vi "Connection Loop.vi"(8 "error in (no error)":errorcluster, 11 "TCP Comm":T2) -> (0 "error out":errorcluster)   [LabVIEW 2020, in "TinyTCP.lvlib"]
uses:
  TinyTCP.lvlib
  Instance.ctl
  Ref Data.ctl
  State.ctl
panel:
  out "Certificate DN":string
  out "TLS Enabled":bool
  out "Server":bool
  out "Port":u16
  out "Host":string
  out "State":T1
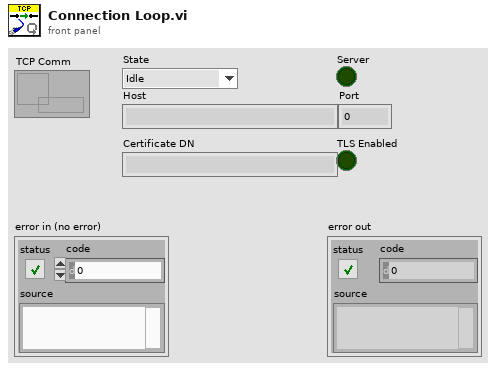
[diagram p1: front panel]
types:
  T1 = typedef "TinyTCP.lvlib/State.ctl" = enum16{"Idle", "Starting", "Connecting", "Connected", "Disconnecting", "Stopped"}
  T2 = typedef "TinyTCP.lvlib/Instance.ctl" = refnum<data-value>
  T3 = typedef "TinyTCP.lvlib/Ref Data.ctl" = cluster{"TCP":refnum<k5>, "State":T1, "Server":bool, "Host":string, "Port":u16, "Listener":refnum<k5>, "Start":bool, "Disconnect":bool, "TCP Valid":bool, "TLS Enabled":bool, "Immutable TLS":refnum<k36>, "Certificate DN":string}
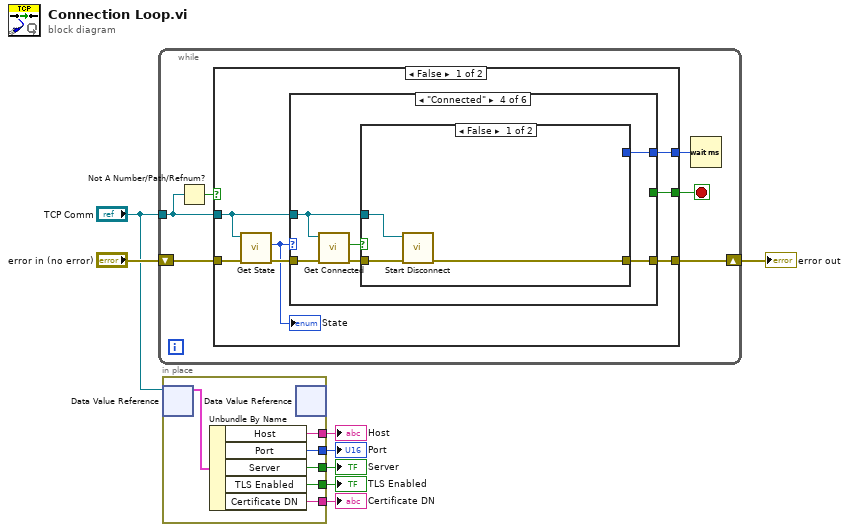
[diagram p0: block diagram]
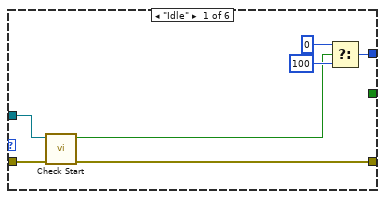
[diagram p2: hidden frame]
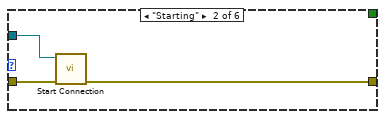
[diagram p3: hidden frame]
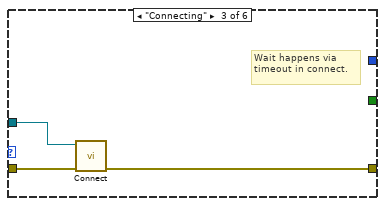
[diagram p4: hidden frame]
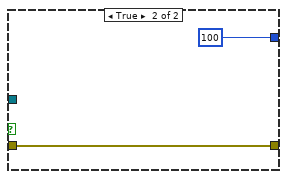
[diagram p5: hidden frame]
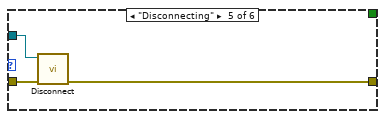
[diagram p6: hidden frame]
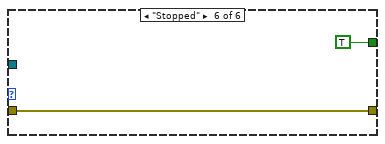
[diagram p7: hidden frame]
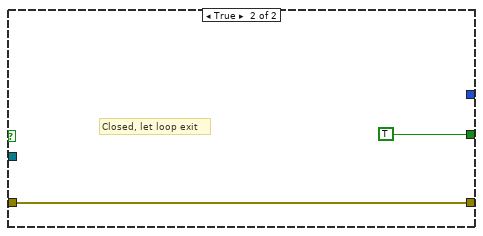
[diagram p8: hidden frame]
diagram:
  n1 = while {
    shift-right: [w9] -> w7
    shift-left: "error in (no error)" -> [w12]
    tunnel: "TCP Comm" -> [w13]
    stop <- w11 stop-if-true
    n2 = Not A Number/Path/Refnum?(number/path/refnum=w13) -> (NaN/Path/Refnum?=w14:bool)
    n3 = case shown="False" w14 {
      tunnel: w13 -> [w19 _]
      tunnel: w12 -> [w18 w51]
      tunnel: [w16 TRUE] -> w11
      tunnel: [w21 _] -> w10
      tunnel: [w20 w51] -> w9
      frame False {
        n4 = call "Get State.vi"("error in (no error)"=w18, "TCP Comm In"=w19) -> ("error out"=w17:errorcluster, "State"=w15:T1)  [unwired: 8 in]
        "State" <- w15
        n5 = case shown="\"Connected\"" w15 {
          tunnel: [w22 _ _ w36 _ _] -> w21
          tunnel: w17 -> [w26 w30 w33 w40 w48 w50]
          tunnel: [w24 w29 w32 w35 w46 w50] -> w20
          tunnel: w19 -> [w25 w31 w34 w37 w47 _]
          tunnel: [_ _ _ _ _ TRUE] -> w16
          frame "Idle" {
            n6 = call "Check Start.vi"("error in (no error)"=w26, "TCP Comm"=w25) -> ("error out"=w24:errorcluster, "Start"=w23:bool)  [unwired: 8 in]
            n7 = Select(t=u32 0 ("milliseconds to wait"), s=w23, f=u32 100 ("milliseconds to wait")) -> (s? t:f=w22:u32)
          }
          frame "Starting" {
            n8 = call "Start Connection.vi"("error in (no error)"=w30, "TCP Comm"=w31) -> ("error out"=w29:errorcluster)  [unwired: 9 in]
          }
          frame "Connecting" {
            # "Wait happens via timeout in connect."
            n9 = call "Connect.vi"("error in (no error)"=w33, "TCP Comm"=w34) -> ("error out"=w32:errorcluster)  [unwired: 9 in]
          }
          frame "Connected" {
            n10 = call "Get Connected.vi"("error in (no error)"=w40, "TCP Comm"=w37) -> ("error out"=w39:errorcluster, "Connected"=w38:bool)  [unwired: 8 in]
            n11 = case shown="False" w38 {
              tunnel: w39 -> [w43 w44]
              tunnel: w37 -> [w42 _]
              tunnel: [_ u32 100 ("milliseconds to wait")] -> w36
              tunnel: [w41 w44] -> w35
              frame False {
                n12 = call "Start Disconnect.vi"("error in (no error)"=w43, "TCP Comm"=w42) -> ("error out"=w41:errorcluster)  [unwired: 9 in]
              }
              frame True {
              }
            }
          }
          frame "Disconnecting" {
            n13 = call "Disconnect.vi"("error in (no error)"=w48, "TCP Comm"=w47) -> ("error out"=w46:errorcluster)  [unwired: 9 in]
          }
          frame "Stopped" {
          }
        }
      }
      frame True {
        # "Closed, let loop exit"
      }
    }
    n14 = Wait (ms)(milliseconds to wait=w10) -> ()  [unwired: 1 out]
  }
  "error out" <- w7
  n15 = in-place {
    in-place-border: [w57] -> w5
    in-place-border: [w56] -> w4
    in-place-border: [w55] -> w3
    in-place-border: [w54] -> w2
    in-place-border: [w53] -> w1
    n16 = in-place-dvr #1("TCP Comm") -> (w58:T3)  [unwired: 1 out]
    n17 = Unbundle By Name(w58) -> ("Host"=w57:string, "Port"=w56:u16, "Server"=w55:bool, "TLS Enabled"=w54:bool, "Certificate DN"=w53:string)
    n18 = in-place-dvr #1() -> ()  [unwired: 1 in, 2 out]
  }
  "Host" <- w5
  "Port" <- w4
  "Server" <- w3
  "TLS Enabled" <- w2
  "Certificate DN" <- w1
